vi "G#Object_RunVI.vi"(0 "vi reference":refnum<vi>, 1 "control names":string[](array[string]), 3 "control values":variant[](array[variant]), 5 "error in (no error)":errorcluster) -> (18 "error out from VI":errorcluster, 19 "error out":errorcluster)   [LabVIEW 2017, in "G#Object.lvclass"]
doc: "Runs the VI specified by the vi reference."
uses:
  G#Object.lvclass
  utils/G#Object_EventType.ctl
  utils/G#Object_ObjectInfoType.ctl
  utils/G#Object_CreateMethod.ctl
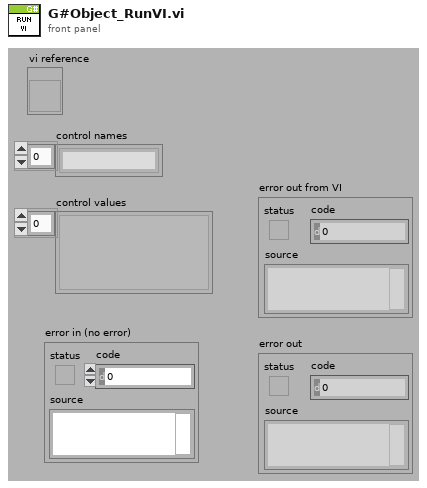
[diagram p1: front panel]
types:
  T1 = typedef "G#Object.lvclass/G#Object_ObjectInfoType.ctl" = cluster{"ObjectName":string, "ObjectID":u32, "Users":i32, "Counter":bool, "AttributeRefs":u32[], "FullClassName":string, "ClassName":string, "CreateMethod":T2, "GenericDestructorExists":bool, "Owner":string}
  T2 = typedef "G#Object.lvclass/G#Object_CreateMethod.ctl" = enum16{"Create", "Create or look up existing", "Look up existing"}
  T3 = typedef "G#Object.lvclass/G#Object_EventType.ctl" = enum16{"Created new", "Looked up existing", "Deleted", "Forced delete", "Not deleted", "Garbage collected", "Cleared", "User", "Error", "External create object", "External create class attributes", "Created class attributes", "Run constructor", "Run constructor done", "Run open method", "Run open method done"}
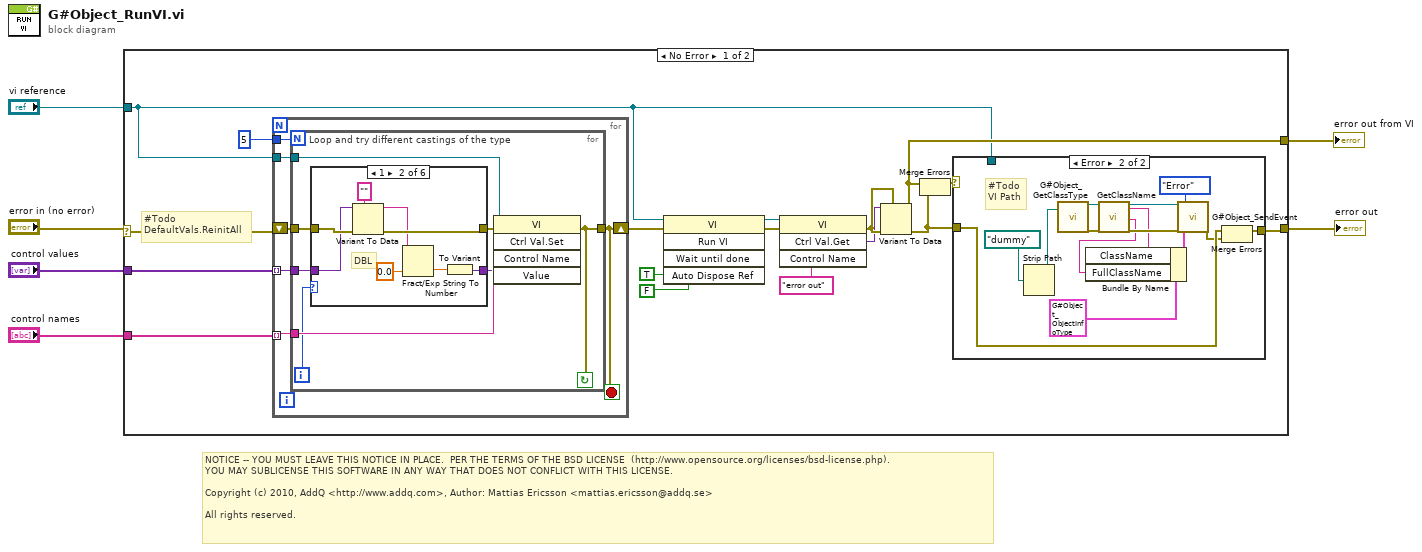
[diagram p0: block diagram]
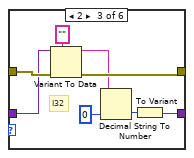
[diagram p4: hidden frame]
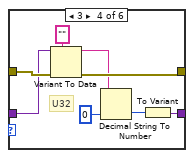
[diagram p5: hidden frame]
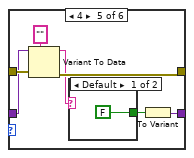
[diagram p6: hidden frame]
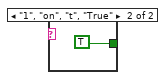
[diagram p7: hidden frame]
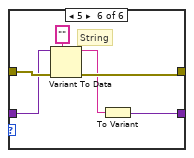
[diagram p8: hidden frame]
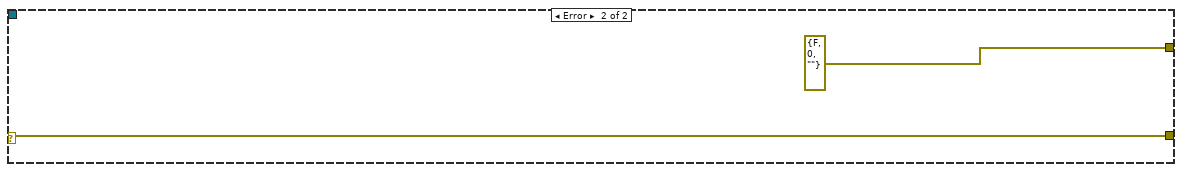
[diagram p9: hidden frame]
diagram:
  # "NOTICE -- YOU MUST LEAVE THIS NOTICE IN PLACE.  PER THE TERMS OF THE BSD LICENSE  (http://www.opensource.org/licenses/bsd-license.php).\nYOU MAY SUBLICENSE THIS SOFTWARE IN ANY WAY THAT DOES NOT CONFLICT WITH THIS LICENSE.\n\nCopyright (c) 2010, AddQ <http://www.addq.com>, Author: Mattias Ericsson <mattias.ericsson@addq.se>\n\nAll rights reserved."
  n1 = case shown="No Error" "error in (no error)" {
    selector: "error in (no error)" -> [w7 w95]
    tunnel: "vi reference" -> [w12 _]
    tunnel: "control values" -> [w19 _]
    tunnel: "control names" -> [w18 _]
    tunnel: [w14 errorcluster {"status"=FALSE, "code"=0, "source"=""} ("error out")] -> w3
    tunnel: [w11 w95] -> w2
    frame No Error {
      # "#Todo\nDefaultVals.ReinitAll"
      n2 = for {
        shift-right: [w39] -> w9
        shift-left: w7 -> [w44]
        tunnel: w12 -> [w43]
        tunnel: w18 -> [w42] mode=indexing
        tunnel: w19 -> [w41] mode=indexing
        tunnel: 5 -> [w40]
        stop <- w39 stop-if-true
        n3 = for {
          N: w40 -> [_]
          tunnel: w44 -> [w47]
          tunnel: w43 -> [w52]
          tunnel: w42 -> [w51]
          tunnel: w41 -> [w49]
          tunnel: [w45] -> w39
          i -> [w50]
          stop <- w45 continue-if-true
          # "Loop and try different castings of the type"
          n4 = case shown="1" w50 {
            tunnel: [w54 w59 w67 w75 w82 w90] -> w48
            tunnel: w49 -> [w54 w61 w69 w77 w84 w92]
            tunnel: w47 -> [w53 w62 w70 w78 w85 w93]
            tunnel: [w53 w60 w68 w76 w83 w91] -> w46
            frame 0, Default {
            }
            frame 1 {
              # "DBL"
              n5 = Variant To Data(error in=w62, type="" ("y"), Variant=w61) -> (data=w57:string, error out=w60:errorcluster)
              n6 = Fract/Exp String To Number(string=w57, default (0 dbl)=0.0 ("default (0 DBL)")) -> (number=w56:dbl)  [unwired: 2 in, 1 out]
              n7 = To Variant(anything=w56) -> (Variant=w59:variant)
            }
            frame 2 {
              # "I32"
              n8 = Variant To Data(error in=w70, type="" ("y"), Variant=w69) -> (data=w65:string, error out=w68:errorcluster)
              n9 = Decimal String To Number(string=w65, default (0L)=0 ("default (0 DBL)")) -> (number=w64:i32)  [unwired: 1 in, 1 out]
              n10 = To Variant(anything=w64) -> (Variant=w67:variant)
            }
            frame 3 {
              # "U32"
              n11 = Variant To Data(error in=w78, type="" ("y"), Variant=w77) -> (data=w73:string, error out=w76:errorcluster)
              n12 = Decimal String To Number(string=w73, default (0L)=u32 0 ("default (0 DBL)")) -> (number=w72:u32)  [unwired: 1 in, 1 out]
              n13 = To Variant(anything=w72) -> (Variant=w75:variant)
            }
            frame 4 {
              n14 = Variant To Data(error in=w85, type="" ("y"), Variant=w84) -> (data=w80:string, error out=w83:errorcluster)
              n15 = case shown="Default" w80 {
                tunnel: [FALSE TRUE] -> w79
                frame Default {
                }
                frame "1", "on", "t", "True" {
                }
              }
              n16 = To Variant(anything=w79) -> (Variant=w82:variant)
            }
            frame 5 {
              # "String"
              n17 = Variant To Data(error in=w93, type="", Variant=w92) -> (data=w88:string, error out=w91:errorcluster)
              n18 = To Variant(anything=w88) -> (Variant=w90:variant)
            }
          }
          n19 = invoke class="VI" method="Ctrl Val.Set"(reference=w52, error in=w46, "Control Name"=w51, "Value"=w48) -> (error out=w45:errorcluster)  [unwired: 1 in, 4 out]
        }
      }
      n20 = invoke class="VI" method="Run VI"(reference=w12, error in=w9, "Wait until done"=TRUE ("Wait Until Done"), "Auto Dispose Ref"=FALSE ("Auto Dispose Reference")) -> (reference out=w20:refnum<vi>, error out=w8:errorcluster)  [unwired: 1 in, 3 out]
      n21 = invoke class="VI" method="Ctrl Val.Get"(reference=w20, error in=w8, "Control Name"="error out") -> (error out=w23:errorcluster, "Get Control Value Variant"=w22:variant)  [unwired: 1 in, 2 out]
      n22 = Variant To Data(error in=w23, type=w23, Variant=w22) -> (data=w14:errorcluster, error out=w10:errorcluster)
      n23 = Merge Errors(w14, w10) -> (w13:errorcluster)
      n24 = case shown="Error" w13 {
        tunnel: w12 -> [_ _]
        tunnel: [w24 w29] -> w11
        tunnel: w10 -> [w24 w28]
        frame No Error {
        }
        frame Error {
          # "#Todo\nVI Path"
          n25 = Strip Path(path=path "dummy") -> (stripped path=w37:path)  [unwired: 1 out]
          n26 = call "G#Object_GetClassType.vi"("class path"=w37) -> ("reference out"=w36:refnum<class "G#Object.lvclass">, "error out"=w35:errorcluster)  [unwired: 17 in]
          n27 = call-dynamic "GetClassName.vi"("reference in"=w36, "error in (no error)"=w35) -> ("reference out"=w34:refnum<class "G#Object.lvclass">, "class name"=w30:string, "full class name"=w26:string, "error out"=w31:errorcluster)  [unwired: 13 in, 1 out]
          n28 = Bundle By Name(cluster=T1 {"ObjectName"="", "ObjectID"=0, "Users"=0, "Counter"=FALSE, "AttributeRefs"=[], "FullClassName"="", "ClassName"="", "CreateMethod"=enum."Create", "GenericDestructorExists"=FALSE, "Owner"=""} ("object info extended"), "ClassName"=w30, "FullClassName"=w26) -> (w32:T1)
          n29 = call "G#Object_SendEvent.vi"("reference in"=w34, "object info extended"=w32, "error in (no error)"=w31, "G# event type"=G#Object_EventType."Error" ("G#Event")) -> ("error out"=w27:errorcluster)  [unwired: 15 in]
          n30 = Merge Errors(w28, w27) -> (w29:errorcluster)
        }
      }
    }
    frame Error {
    }
  }
  "error out" <- w2
  "error out from VI" <- w3
